vi "GetUhpCaptureMode.vi"(0 "Camera Reference in":refnum<k24>, 1 "error in (no error)":errorcluster) -> (2 "Camera Reference out":refnum<k24>, 3 "error out":errorcluster, 4 "UhpCaptureMode (Camera1 Camera2 Merge)":u8(ring) items=["Camera1", "Camera2", "Merge"])   [LabVIEW 2023]
uses:
  C:/Mech-Mind/Mech-Eye SDK-2.5.0-b5-dev-01-03/API/dll/net48/MechEyeApiNet.dll
  dll/net48/MechEyeApiNet.dll
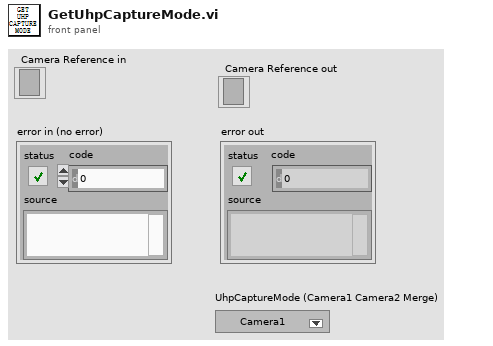
[diagram p1: front panel]
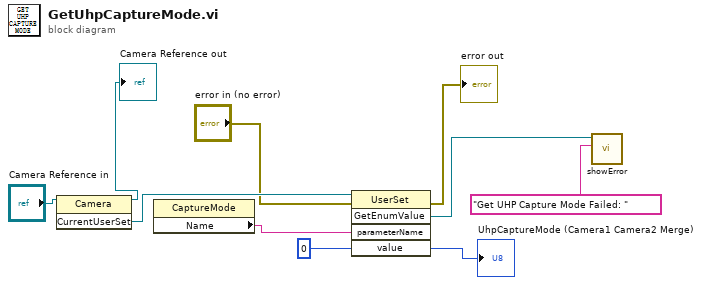
[diagram p0: block diagram]
diagram:
  n1 = invoke class="Camera" method="CurrentUserSet"(reference="Camera Reference in") -> (reference out=→"Camera Reference out":refnum<k24>, "CurrentUserSet"=w4:refnum<k24>)  [unwired: 2 in, 1 out]
  n2 = property class="CaptureMode"() -> ("Name"=w8:string)  [unwired: 2 in, 2 out]
  n3 = invoke class="UserSet" method="GetEnumValue"(reference=w4, error in="error in (no error)", "parameterName"=w8, "value"=0) -> (error out=→"error out":errorcluster, "GetEnumValue"=w5:refnum<k24>, "value"=→"UhpCaptureMode (Camera1 Camera2 Merge)":i32)  [unwired: 1 in, 2 out]
  n4 = call "showError.vi"("String"="Get UHP Capture Mode Failed: ", "MMind.Eye.ErrorStatus"=w5) -> ()  [unwired: 10 in]
